vi "NI CardSelfTest.vi"(8 "error in":errorcluster) -> (0 "error out":errorcluster, 2 "Report Text":string, 3 "OK":bool)   [LabVIEW 2023, in "LTT_TeststandSteptypes.lvlib"]
uses:
  LTT_TeststandSteptypes.lvlib
  HardwareAbstractionLayer_LVOOP/Database/Database.lvclass
  HardwareAbstractionLayer_LVOOP/Database/SQL Public VI/Control/DB Options.ctl
  <userlib>/_OpenG.lib/error/error.llb/openg_error.lvlib
panel:
  out "NIFGENSelfTest":bool[](array[boolean])
  out "NIDMMSelfTest":bool[](array[boolean])
  out "NIScopeSelfTest":bool[](array[boolean])
  out "NIRelaySelfTest":bool[](array[boolean])
  out "NI DAQ Self Test":bool[](array[boolean])
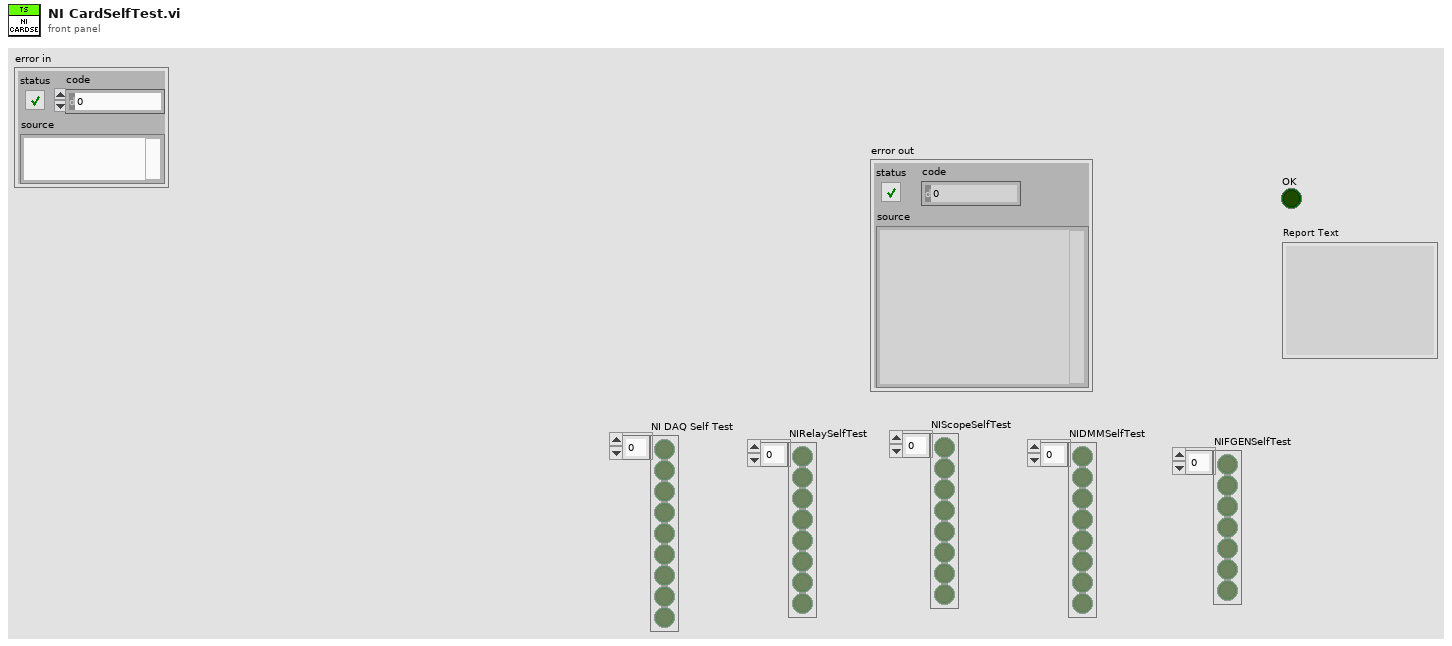
[diagram p1: front panel]
types:
  T1 = typedef "HardwareAbstractionLayer_LVOOP.lvlib/Database.lvclass/DB Options.ctl" = enum16{"Init", "Select Data", "Insert Data", "Update Data", "Delete Data", "Execute Query", "Create Schema", "Create Table", "List Tables", "List Columns", "Close"}
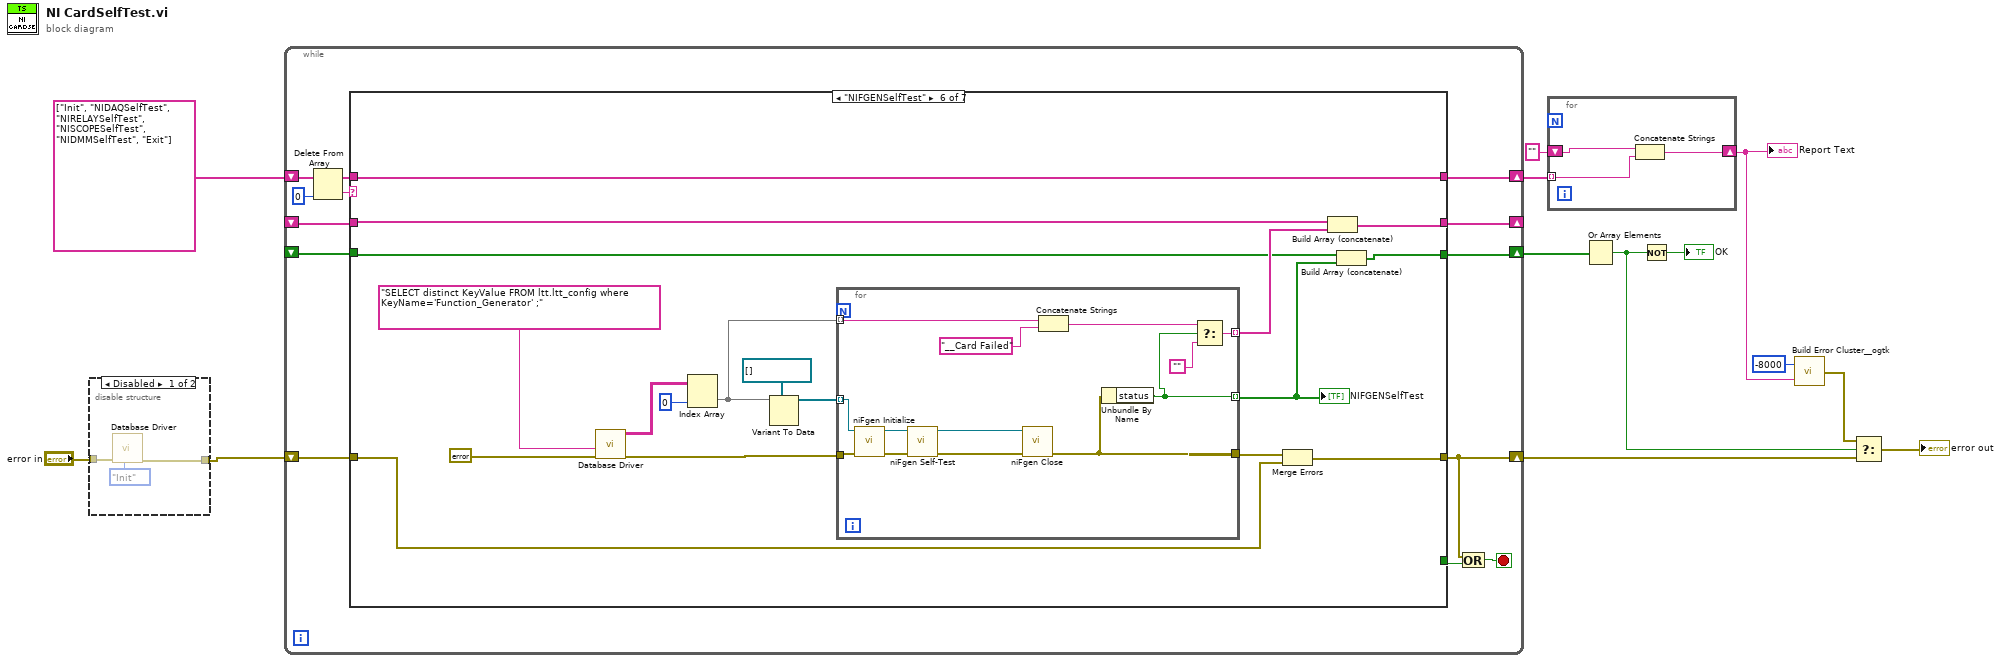
[diagram p0: block diagram]
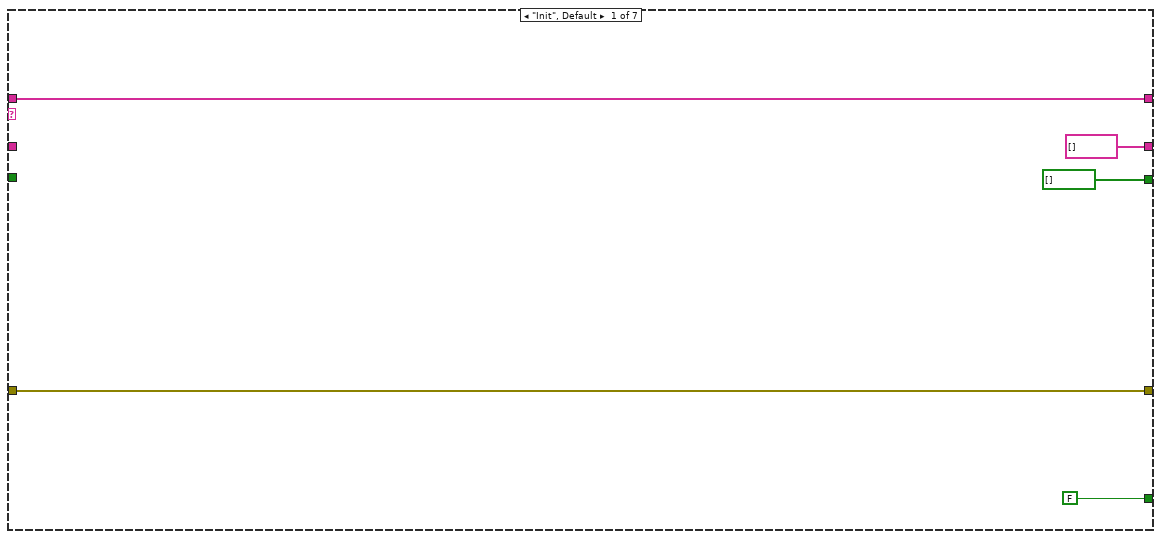
[diagram p2: hidden frame]
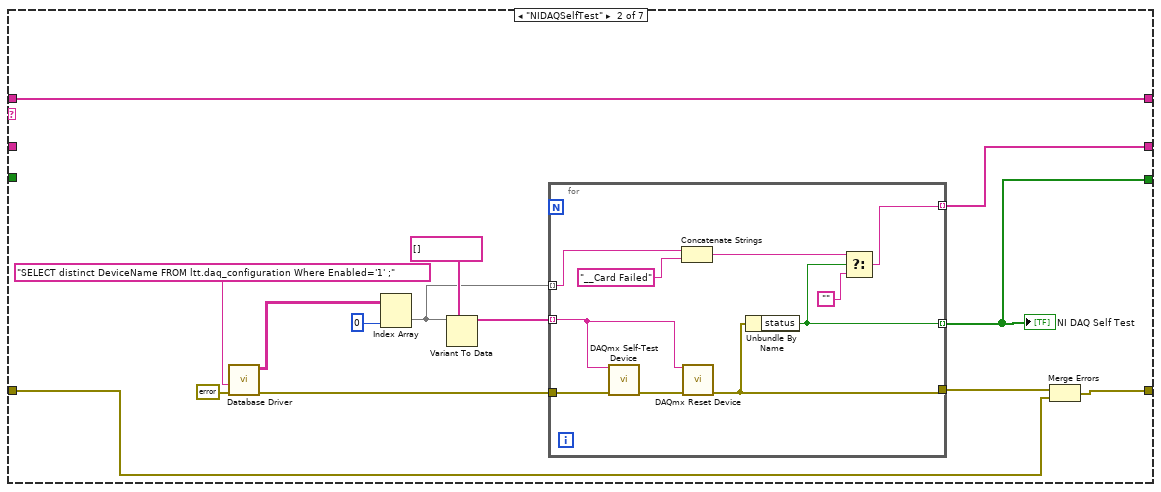
[diagram p3: hidden frame]
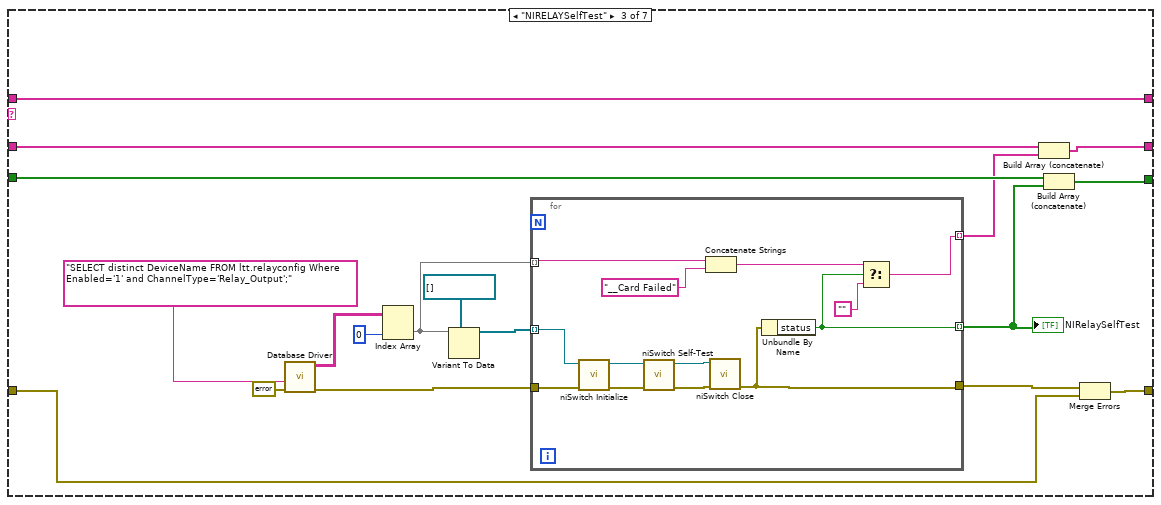
[diagram p4: hidden frame]
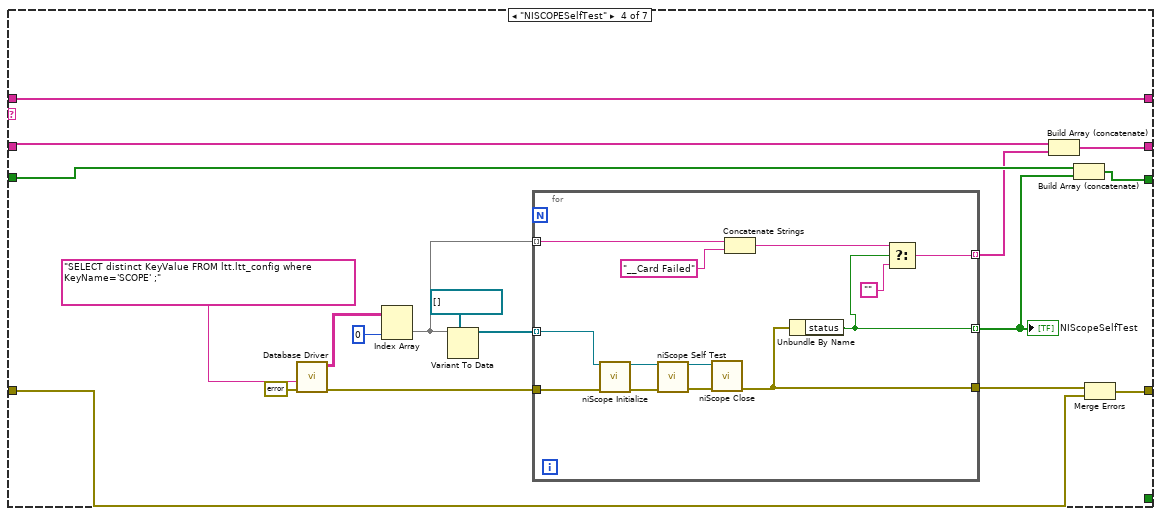
[diagram p5: hidden frame]
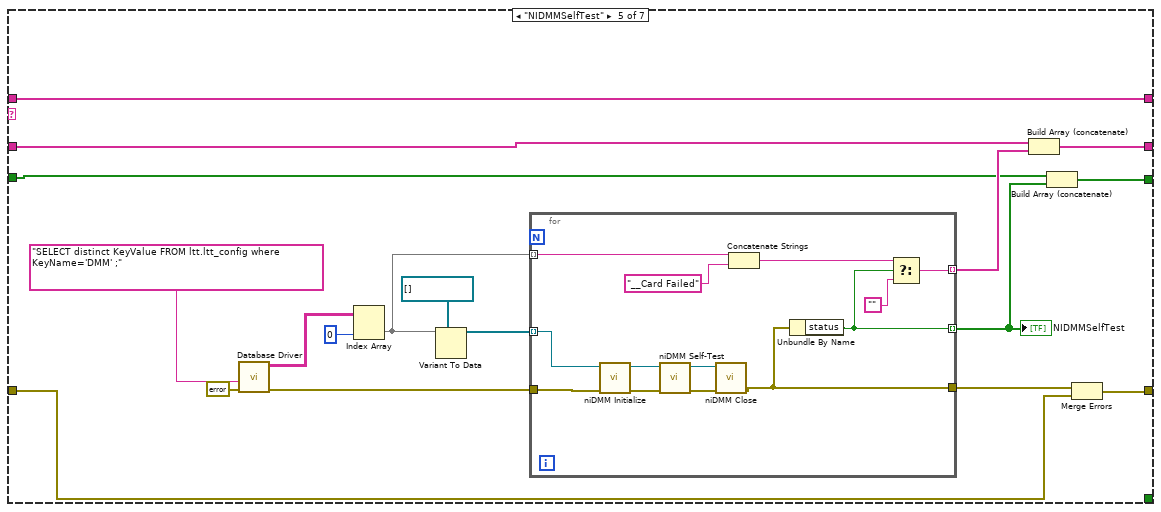
[diagram p6: hidden frame]
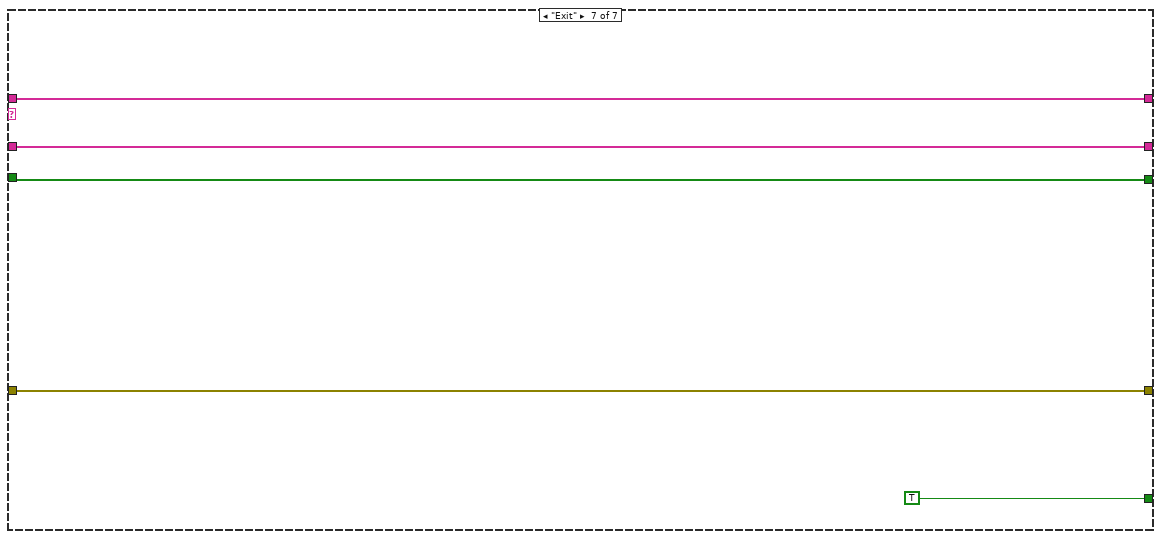
[diagram p7: hidden frame]
diagram:
  n1 = disable-structure shown="Disabled" {
    disable-tunnel: "error in" -> [w15 w17]
    disable-tunnel: [w14 w17] -> w12
    frame Disabled {
      n2 = call "Database Driver.vi"("Options"=DB_Options."Init", "error in"=w15) -> ("error out"=w14:errorcluster)  [unwired: 6 in, 3 out]
    }
    frame Enabled {
    }
  }
  n3 = while {
    shift-right: [w19] -> w4
    shift-left: w12 -> [w30]
    shift-right: [w25] -> w9
    shift-left: string[] ["Init", "NIDAQSelfTest", "NIRELAYSelfTest", "NISCOPESelfTest", "NIDMMSelfTest", "Exit"] -> [w29]
    shift-right: [w21] -> w10
    shift-left: _ -> [w24]
    shift-right: [w23] -> _
    shift-left: _ -> [w22]
    stop <- w20 stop-if-true
    n4 = Delete From Array(array=w29, index=0) -> (deleted portion=w27:string, array with subset deleted=w26:string[])  [unwired: 1 in]
    n5 = case shown="\"NIFGENSelfTest\"" w27 {
      tunnel: w30 -> [w35 w38 w67 w98 w129 w160 w188]
      tunnel: [w35 w39 w68 w99 w130 w161 w188] -> w19
      tunnel: [w34 w41 w70 w102 w133 w164 w187] -> w25
      tunnel: w26 -> [w34 w41 w70 w102 w133 w164 w187]
      tunnel: [FALSE _ _ _ _ _ TRUE] -> w18
      tunnel: w24 -> [_ _ w65 w96 w124 w155 w184]
      tunnel: [string[] [] w37 w61 w93 w125 w157 w185] -> w23
      tunnel: w22 -> [_ _ w63 w94 w126 w158 w185]
      tunnel: [bool[] [] w36 w60 w91 w122 w153 w184] -> w21
      frame "Init", Default {
      }
      frame "NIDAQSelfTest" {
        n6 = call "Database Driver.vi"("error in"=errorcluster {"status"=FALSE, "code"=0, "source"=""}, "SQL query"="SELECT distinct DeviceName FROM ltt.daq_configuration Where Enabled='1' ;") -> ("error out"=w46:errorcluster, "data"=w47:string[][])  [unwired: 6 in, 2 out]
        n7 = Index Array(array=w47, index (col)=0 ("disabled index (col)")) -> (element=w44:string[])  [unwired: 1 in]
        n8 = Variant To Data(type=tag[] [] ("DeviceName"), Variant=w44) -> (data=w45:tag[])  [unwired: 1 in, 1 out]
        n9 = for {
          tunnel: w46 -> [w59]
          tunnel: w45 -> [w57] mode=indexing
          tunnel: w44 -> [w54] mode=indexing
          tunnel: [w56] -> w42
          tunnel: [w55] -> w36 mode=indexing
          tunnel: [w50] -> w37 mode=indexing
          n10 = call <vilib>:"DAQmx Self-Test Device.vi"("device in"=w57, "error in"=w59) -> ("error out"=w58:errorcluster)  [unwired: 13 in]
          n11 = Concatenate Strings(w54, "__Card Failed" ("string")) -> (w52:string)
          n12 = call <vilib>:"DAQmx Reset Device.vi"("device in"=w57, "error in"=w58) -> ("error out"=w56:errorcluster)  [unwired: 13 in]
          n13 = Unbundle By Name(w56) -> ("status"=w55:bool)
          n14 = Select(t=w52, s=w55, f="") -> (s? t:f=w50:string)
        }
        "NI DAQ Self Test" <- w36
        n15 = Merge Errors(w42, w38) -> (w39:errorcluster)
      }
      frame "NIRELAYSelfTest" {
        n16 = call "Database Driver.vi"("error in"=errorcluster {"status"=FALSE, "code"=0, "source"=""}, "SQL query"="SELECT distinct DeviceName FROM ltt.relayconfig Where Enabled='1' and ChannelType='Relay_Output';") -> ("error out"=w77:errorcluster, "data"=w75:string[][])  [unwired: 6 in, 2 out]
        n17 = Index Array(array=w75, index (col)=0 ("disabled index (col)")) -> (element=w66:string[])  [unwired: 1 in]
        n18 = Variant To Data(type=refnum<k15>[] [], Variant=w66) -> (data=w76:refnum<k15>[])  [unwired: 1 in, 1 out]
        n19 = for {
          tunnel: w76 -> [w90] mode=indexing
          tunnel: w77 -> [w89]
          tunnel: [w80] -> w64 mode=indexing
          tunnel: [w85] -> w71
          tunnel: w66 -> [w79] mode=indexing
          tunnel: [w78] -> w62 mode=indexing
          n20 = call <instrlib>:"niSwitch Initialize.vi"("error in (no error)"=w89, "resource name"=w90) -> ("error out"=w87:errorcluster, "instrument handle out"=w88:refnum<k15>)  [unwired: 8 in]
          n21 = call <instrlib>:"niSwitch Self-Test.vi"("error in (no error)"=w87, "instrument handle"=w88) -> ("error out"=w86:errorcluster, "instrument handle out"=w84:refnum<k15>)  [unwired: 6 in, 2 out]
          n22 = Concatenate Strings(w79, "__Card Failed" ("string")) -> (w82:string)
          n23 = call <instrlib>:"niSwitch Close.vi"("error in (no error)"=w86, "instrument handle"=w84) -> ("error out"=w85:errorcluster)  [unwired: 9 in]
          n24 = Unbundle By Name(w85) -> ("status"=w80:bool)
          n25 = Select(t=w82, s=w80, f="") -> (s? t:f=w78:string)
        }
        "NIRelaySelfTest" <- w64
        n26 = Build Array (concatenate)(w63, w62) -> (w61:string[])
        n27 = Build Array (concatenate)(w65, w64) -> (w60:bool[])
        n28 = Merge Errors(w71, w67) -> (w68:errorcluster)
      }
      frame "NISCOPESelfTest" {
        n29 = call "Database Driver.vi"("error in"=errorcluster {"status"=FALSE, "code"=0, "source"=""}, "SQL query"="SELECT distinct KeyValue FROM ltt.ltt_config where KeyName='SCOPE' ;") -> ("error out"=w108:errorcluster, "data"=w106:string[][])  [unwired: 6 in, 2 out]
        n30 = Index Array(array=w106, index (col)=0 ("disabled index (col)")) -> (element=w97:string[])  [unwired: 1 in]
        n31 = Variant To Data(type=refnum<k15>[] [], Variant=w97) -> (data=w107:refnum<k15>[])  [unwired: 1 in, 1 out]
        n32 = for {
          tunnel: w107 -> [w119] mode=indexing
          tunnel: w108 -> [w121]
          tunnel: [w111] -> w95 mode=indexing
          tunnel: [w115] -> w103
          tunnel: w97 -> [w110] mode=indexing
          tunnel: [w109] -> w92 mode=indexing
          n33 = call <instrlib>:"niScope Initialize.vi"("resource name"=w119, "error in"=w121) -> ("instrument handle"=w118:refnum<k15>, "error out"=w120:errorcluster)  [unwired: 12 in]
          n34 = call <instrlib>:"niScope Self Test.vi"("instrument handle"=w118, "error in"=w120) -> ("instrument handle out"=w117:refnum<k15>, "error out"=w116:errorcluster)  [unwired: 10 in, 2 out]
          n35 = call <instrlib>:"niScope Close.vi"("instrument handle"=w117, "error in"=w116) -> ("error out"=w115:errorcluster)  [unwired: 13 in]
          n36 = Concatenate Strings(w110, "__Card Failed" ("string")) -> (w113:string)
          n37 = Unbundle By Name(w115) -> ("status"=w111:bool)
          n38 = Select(t=w113, s=w111, f="") -> (s? t:f=w109:string)
        }
        "NIScopeSelfTest" <- w95
        n39 = Build Array (concatenate)(w94, w92) -> (w93:string[])
        n40 = Build Array (concatenate)(w96, w95) -> (w91:bool[])
        n41 = Merge Errors(w103, w98) -> (w99:errorcluster)
      }
      frame "NIDMMSelfTest" {
        n42 = call "Database Driver.vi"("error in"=errorcluster {"status"=FALSE, "code"=0, "source"=""}, "SQL query"="SELECT distinct KeyValue FROM ltt.ltt_config where KeyName='DMM' ;") -> ("error out"=w139:errorcluster, "data"=w137:string[][])  [unwired: 6 in, 2 out]
        n43 = Index Array(array=w137, index (col)=0 ("disabled index (col)")) -> (element=w128:string[])  [unwired: 1 in]
        n44 = Variant To Data(type=refnum<k15>[] [], Variant=w128) -> (data=w138:refnum<k15>[])  [unwired: 1 in, 1 out]
        n45 = for {
          tunnel: w138 -> [w147] mode=indexing
          tunnel: w139 -> [w152]
          tunnel: [w140] -> w123 mode=indexing
          tunnel: [w149] -> w134
          tunnel: w128 -> [w142] mode=indexing
          tunnel: [w141] -> w127 mode=indexing
          n46 = call <instrlib>:"niDMM Initialize.vi"("error in (no error)"=w152, "Instrument Descriptor"=w147) -> ("error out"=w148:errorcluster, "instrument handle out"=w146:refnum<k15>)  [unwired: 8 in]
          n47 = call <instrlib>:"niDMM Self-Test.vi"("error in (no error)"=w148, "instrument handle"=w146) -> ("error out"=w151:errorcluster, "instrument handle out"=w150:refnum<k15>)  [unwired: 6 in, 2 out]
          n48 = call <instrlib>:"niDMM Close.vi"("error in (no error)"=w151, "instrument handle"=w150) -> ("error out"=w149:errorcluster)  [unwired: 9 in]
          n49 = Concatenate Strings(w142, "__Card Failed" ("string")) -> (w144:string)
          n50 = Unbundle By Name(w149) -> ("status"=w140:bool)
          n51 = Select(t=w144, s=w140, f="") -> (s? t:f=w141:string)
        }
        "NIDMMSelfTest" <- w123
        n52 = Build Array (concatenate)(w126, w127) -> (w125:string[])
        n53 = Build Array (concatenate)(w124, w123) -> (w122:bool[])
        n54 = Merge Errors(w134, w129) -> (w130:errorcluster)
      }
      frame "NIFGENSelfTest" {
        n55 = call "Database Driver.vi"("error in"=errorcluster {"status"=FALSE, "code"=0, "source"=""}, "SQL query"="SELECT distinct KeyValue FROM ltt.ltt_config where KeyName='Function_Generator' ;") -> ("error out"=w170:errorcluster, "data"=w168:string[][])  [unwired: 6 in, 2 out]
        n56 = Index Array(array=w168, index (col)=0 ("disabled index (col)")) -> (element=w159:string[])  [unwired: 1 in]
        n57 = Variant To Data(type=refnum<k15>[] [], Variant=w159) -> (data=w169:refnum<k15>[])  [unwired: 1 in, 1 out]
        n58 = for {
          tunnel: w169 -> [w182] mode=indexing
          tunnel: w170 -> [w181]
          tunnel: [w173] -> w154 mode=indexing
          tunnel: [w177] -> w165
          tunnel: w159 -> [w172] mode=indexing
          tunnel: [w171] -> w156 mode=indexing
          n59 = call <instrlib>:"niFgen Initialize.vi"("error in (no error)"=w181, "Resource Name"=w182) -> ("error out"=w180:errorcluster, "Instrument Handle Out"=w179:refnum<k15>)  [unwired: 8 in]
          n60 = call <instrlib>:"niFgen Self-Test.vi"("error in (no error)"=w180, "Instrument Handle"=w179) -> ("error out"=w183:errorcluster, "Instrument Handle Out"=w178:refnum<k15>)  [unwired: 6 in, 2 out]
          n61 = call <instrlib>:"niFgen Close.vi"("error in (no error)"=w183, "Instrument Handle"=w178) -> ("error out"=w177:errorcluster)  [unwired: 9 in]
          n62 = Concatenate Strings(w172, "__Card Failed" ("string")) -> (w175:string)
          n63 = Unbundle By Name(w177) -> ("status"=w173:bool)
          n64 = Select(t=w175, s=w173, f="") -> (s? t:f=w171:string)
        }
        "NIFGENSelfTest" <- w154
        n65 = Merge Errors(w165, w160) -> (w161:errorcluster)
        n66 = Build Array (concatenate)(w158, w156) -> (w157:string[])
        n67 = Build Array (concatenate)(w155, w154) -> (w153:bool[])
      }
      frame "Exit" {
      }
    }
    n68 = Compound Arithmetic op=OR(w19, w18) -> (w20:bool)
  }
  n69 = for {
    tunnel: w9 -> [w191] mode=indexing
    shift-right: [w190] -> w6
    shift-left: "" -> [w189]
    n70 = Concatenate Strings(w189, w191) -> (w190:string)
  }
  "Report Text" <- w6
  n71 = Or Array Elements(Boolean array=w10) -> (logical OR=w5:bool)
  n72 = Not(x=w5) -> (.not. x?=→"OK":bool)
  n73 = call <userlib>:"Build Error Cluster__ogtk.vi"("String to Prepend to source (\"\")"=w6, "code"=-8000) -> ("error out"=w8:errorcluster)
  n74 = Select(t=w8, s=w5, f=w4) -> (s? t:f=→"error out":errorcluster)
